vi "ColorDetection2 (2).vi"() -> ()   [LabVIEW 2018]
uses:
  Control 1.ctl
  <vilib>/myRIO/Instrument Drivers/Onboard IO/DIO/typedefs/DIO Reference.ctl
  <vilib>/myRIO/Common/Instrument Driver Framework/Utilities/typedefs/myRIO Generic Hardware Reference.ctl
  <vilib>/myRIO/Common/Instrument Driver Framework/Utilities/typedefs/Hardware Version Enum.ctl
  <vilib>/myRIO/Common/Instrument Driver Framework/Utilities/typedefs/myRIO v1.0 Reference.ctl
  <vilib>/myRIO/Common/Instrument Driver Framework/Utilities/typedefs/Generic FPGA Reference.ctl
  <vilib>/myRIO/Common/Instrument Driver Framework/myRIO v1.0/DIO/typedefs/DIO Channels List.ctl
  <vilib>/myRIO/Common/Instrument Driver Framework/myRIO v1.0/DIO/typedefs/DIO Channels Enum.ctl
  <vilib>/userdefined/High Color/nirio_resource_hc.ctl
  <vilib>/myRIO/Common/Instrument Driver Framework/Utilities/vis/Is FPGA Ref Available.vi
  <vilib>/myRIO/Common/Instrument Driver Framework/myRIO v1.0/DIO/vis/myRIO v1.1 Open DIO.vi
  <vilib>/myRIO/Instrument Drivers/Onboard IO/DIO/vis/Write.vi
  <vilib>/myRIO/Common/Instrument Driver Framework/Utilities/vis/Validate Channels.vi
  <vilib>/myRIO/Common/Instrument Driver Framework/myRIO v1.0/DIO/vis/myRIO v1.0 Reserve DIO.vi
  <vilib>/myRIO/Common/Instrument Driver Framework/myRIO v1.0/UART/vis/myRIO v1.0 Close UART.vi
  <vilib>/myRIO/Common/Instrument Driver Framework/myRIO v1.0/Resource Manager/vis/myRIO v1.0 Reserve Channel List.vi
  <vilib>/myRIO/Common/Instrument Driver Framework/myRIO v1.0/DIO/vis/myRIO v1.0 Build MUX Configuration DIO.vi
  <vilib>/myRIO/Common/Instrument Driver Framework/myRIO v1.0/Resource Manager/vis/myRIO v1.0 Reserve Channel.vi
  <vilib>/myRIO/Common/Instrument Driver Framework/myRIO v1.0/Resource Manager/vis/myRIO v1.0 Unreserve Channel.vi
  <vilib>/myRIO/Common/Instrument Driver Framework/myRIO v1.0/Resource Manager/vis/myRIO v1.0 Create Configuration List.vi
  <vilib>/myRIO/Common/Instrument Driver Framework/myRIO v1.0/Resource Manager/vis/myRIO v1.0 Build Mutex Name.vi
  <vilib>/Utility/VariantDataType/GetNumericInfo.vi
  <vilib>/Utility/error.llb/Error Cluster From Error Code.vi
  <vilib>/myRIO/Common/Instrument Driver Framework/myRIO v1.0/myRIO v1.1 Open.vi
  <vilib>/myRIO/Common/Instrument Driver Framework/Utilities/vis/IO Manager.vi
  <vilib>/myRIO/Common/Instrument Driver Framework/Utilities/vis/Configuration Manager.vi
  <vilib>/myRIO/Common/Instrument Driver Framework/myRIO v1.0/Resource Manager/vis/myRIO v1.0 Configure IO.vi
  <vilib>/myRIO/Common/Instrument Driver Framework/myRIO v1.0/myRIO v1.0 Close.vi
  <vilib>/myRIO/Common/Instrument Driver Framework/myRIO v1.0/DIO/vis/myRIO v1.0 Write DIO.vi
  <vilib>/myRIO/Common/Instrument Driver Framework/Utilities/vis/FPGA Ref Manager.vi
  <vilib>/myRIO/Common/Instrument Driver Framework/myRIO v1.0/myRIO v1.0 Reset FPGA.vi
  <vilib>/myRIO/Common/Instrument Driver Framework/myRIO v1.0/IRQ/vis/myRIO v1.0 IRQ Info FGV.vi
  <vilib>/myRIO/Common/Instrument Driver Framework/myRIO v1.0/IRQ/vis/myRIO v1.0 Timer IRQ Info FGV.vi
  <vilib>/myRIO/Common/Instrument Driver Framework/myRIO v1.0/IRQ/vis/myRIO v1.0 ISR Agent.vi
  <vilib>/myRIO/Express VI/Onboard IO/DO/DO Express VI.xnode
  <vilib>/myRIO/Instrument Drivers/Onboard IO/DIO/vis/myRIO DIO Open.xnode
  <vilib>/myRIO/Instrument Drivers/Utilities/Utilities.lvlib
  <vilib>/myRIO/Instrument Drivers/Onboard IO/DIO/DIO.lvlib
panel:
  out "Time has Elapsed 8":bool caption="Time has Elapsed"
  out "Time has Elapsed 7":bool caption="Time has Elapsed"
  out "Time has Elapsed 6":bool caption="Time has Elapsed"
  out "Time has Elapsed 5":bool caption="Time has Elapsed"
  out "Time has Elapsed 4":bool caption="Time has Elapsed"
  out "Amarillo":bool
  out "Rojo":bool
  out "Azul":bool
  out "Verde":bool
  out "Time has Elapsed 3":bool caption="Time has Elapsed"
  out "Time has Elapsed 2":bool caption="Time has Elapsed"
  out "Time has Elapsed":bool
  out "Negro 3":bool
  out "Amarillo 3":bool
  out "Rojo 3":bool
  out "Azul 3":bool
  out "Verde 3":bool
  out "Color Spectrum 7":dbl[](array[numeric]) format="%.2f"
  out "h3":bool
  out "h2":bool
  out "h1":bool
  out "h0":bool
  out "Negro 1":bool
  out "Amarillo 1":bool
  out "Rojo 1":bool
  out "Azul 1":bool
  out "Verde 1":bool
  out "Negro 2":bool
  out "Amarillo 2":bool
  out "Rojo 2":bool
  out "Azul 2":bool
  out "Verde 2":bool
  out "Color Spectrum 6":dbl[](array[numeric]) format="%.2f"
  out "Color Spectrum 5":dbl[](array[numeric]) format="%.2f"
  out "Negro":bool
  out "Amarillo":bool
  out "Rojo":bool
  out "Azul":bool
  out "Verde":bool
  out "Image Out":T1(plugin-control)
  out "Color Spectrum 4":dbl[](array[numeric]) format="%.2f"
  in  "Stop (F) 2":bool caption="Stop (F)"
  out "Estados":T2
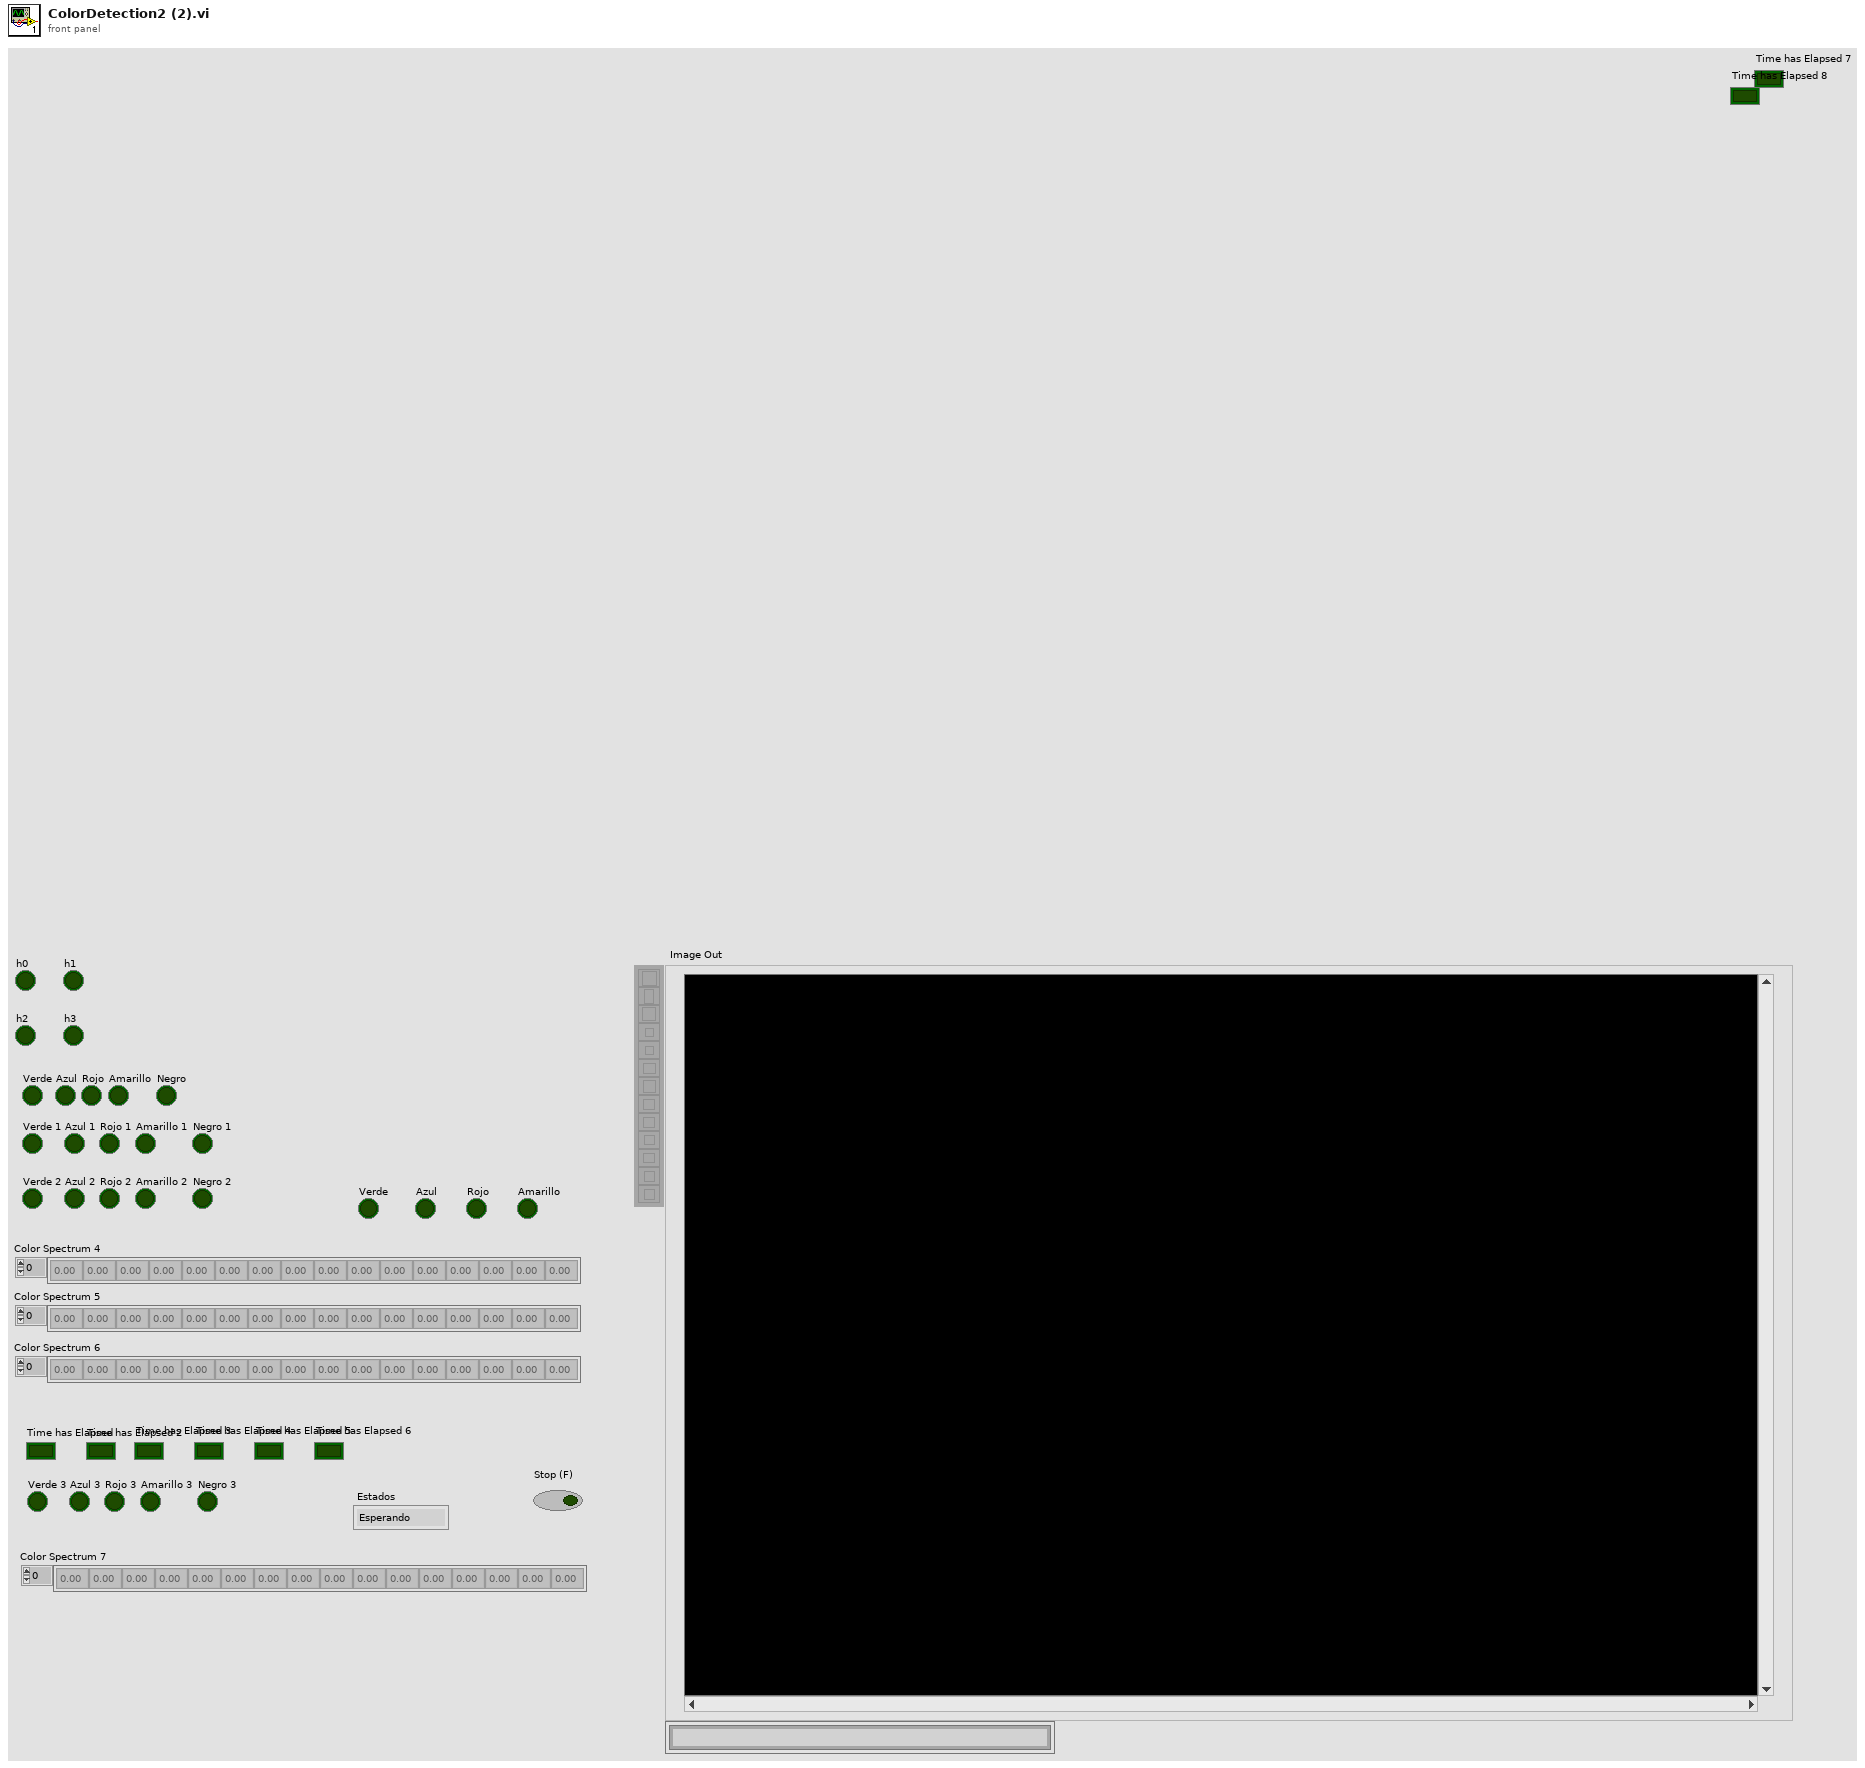
[diagram p1: front panel]
types:
  T1 = typedef "IMAQ Image.ctl" = refnum<image>
  T2 = typedef "Control 1.ctl" = enum16{"Esperando", "Seccion1", "Seccion2", "Seccion3", "Seccion4", "Seccion5", "Seccion6", "Seccion7", "Seccion8", "Seccion9", "Seccion10", "Seccion11", "Seccion12"}
  T3 = typedef "IMAQ Rectangle" = cluster{"Left":i32, "Top":i32, "Right":i32, "Bottom":i32, "Rotation":dbl}
  T4 = typedef "DIO.lvlib/DIO Reference.ctl" = cluster{"myRIO Reference":T5, "DIO Channels List":T9}
  T5 = typedef "myRIO Generic Hardware Reference.ctl" = cluster{"myRIO Model":T6, "myRIO Hardware Reference":T7}
  T6 = typedef "Hardware Version Enum.ctl" = enum16{"Unknown", "myRIO-1900", "myRIO-1950", "roboRIO", "NI ELVIS RIO CM", "ELVIS III"}
  T7 = typedef "myRIO v1.0 Reference.ctl" = cluster{"Generic FPGA Reference":T8, "Allow multiple opens":bool}
  T8 = typedef "Generic FPGA Reference.ctl" = refnum<k20>
  T9 = typedef "DIO Channels List.ctl" = T10[]
  T10 = typedef "DIO Channels Enum.ctl" = enum16{"Not Connected", "C/DIO0", "C/DIO1", "C/DIO2", "C/DIO3", "C/DIO4", "C/DIO5", "C/DIO6", "C/DIO7", "A/DIO0", "A/DIO1", "A/DIO2", "A/DIO3", "A/DIO4", "A/DIO5", "A/DIO6", "A/DIO7", "A/DIO8", "A/DIO9", "A/DIO10", "A/DIO11", "A/DIO12", "A/DIO13", "A/DIO14", "A/DIO15", "A/DIO16", "A/DIO17", "A/DIO18", "A/DIO19", "B/DIO0", "B/DIO1", "B/DIO2", "B/DIO3", "B/DIO4", "B/DIO5", "B/DIO6", "B/DIO7", "B/DIO8", "B/DIO9", "B/DIO10", "B/DIO11", "B/DIO12", "B/DIO13", "B/DIO14", "B/DIO15", "B/DIO16", "B/DIO17", "B/DIO18", "B/DIO19", "LED0", "LED1", "LED2", "LED3", "Button0", "DIO/DIO0", "DIO/DIO1", "DIO/DIO2", "DIO/DIO3", "DIO/DIO4", "DIO/DIO5", "DIO/DIO6", "DIO/DIO7", "DIO/DIO8", "DIO/DIO9", "SPI/CS0", "SPI/CS1", "SPI/CS2", "SPI/CS3", "LED RADIO (Green)", "LED RADIO (Red)", "LED COMM (Green)", "LED COMM (Red)", "LED MODE (Green)", "LED MODE (Red)"}
  T11 = typedef "nirio_resource_hc.ctl" = tag
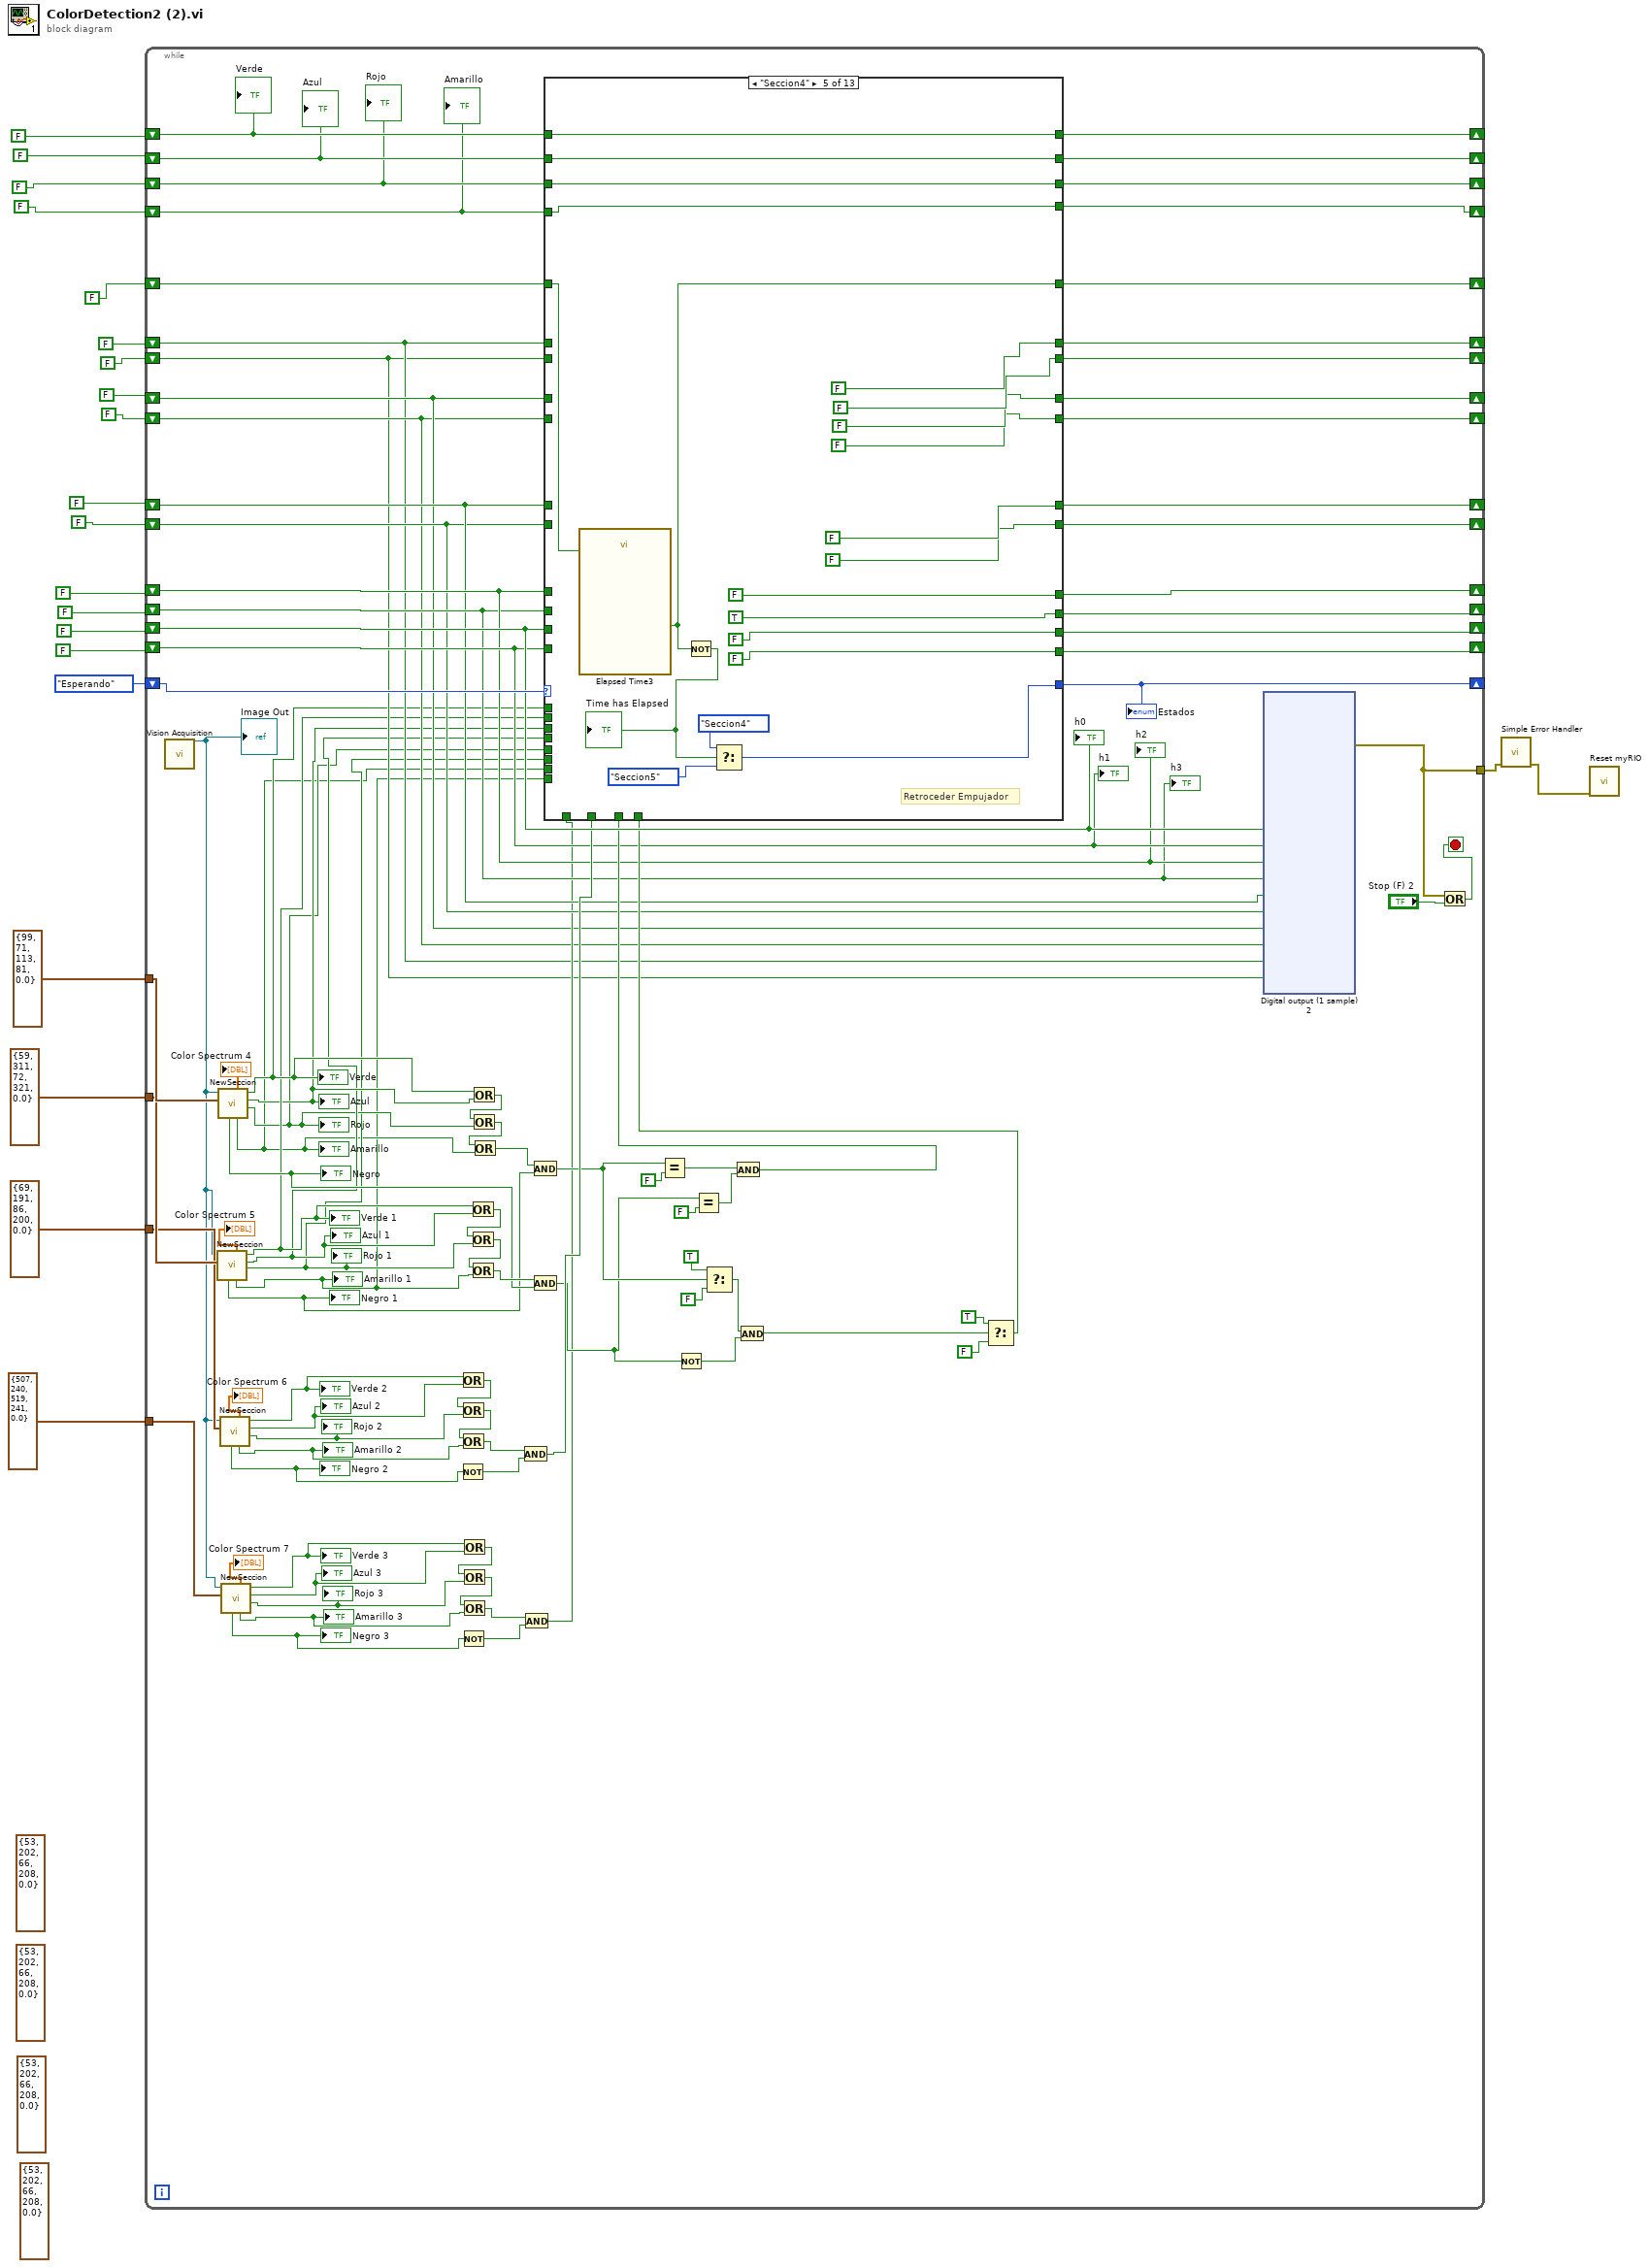
[diagram p0: block diagram]
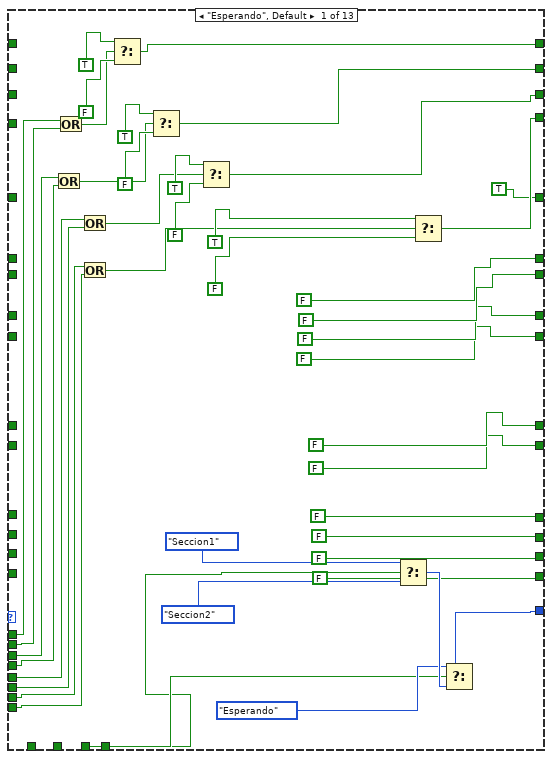
[diagram p2: hidden frame]
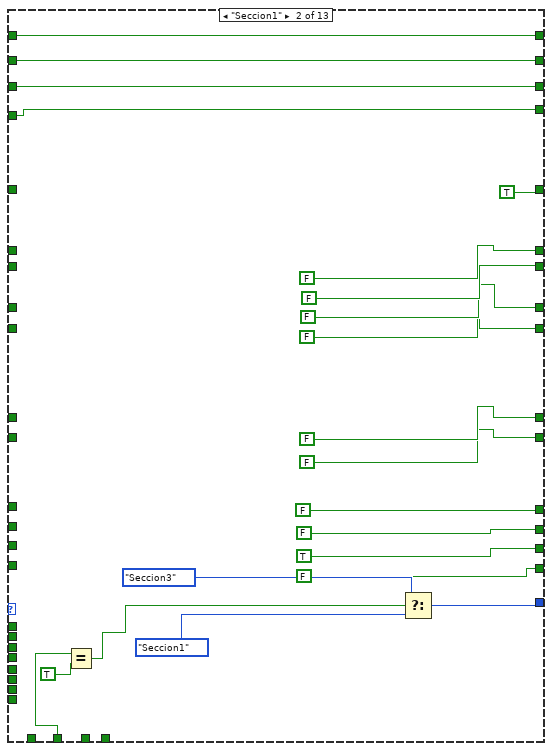
[diagram p3: hidden frame]
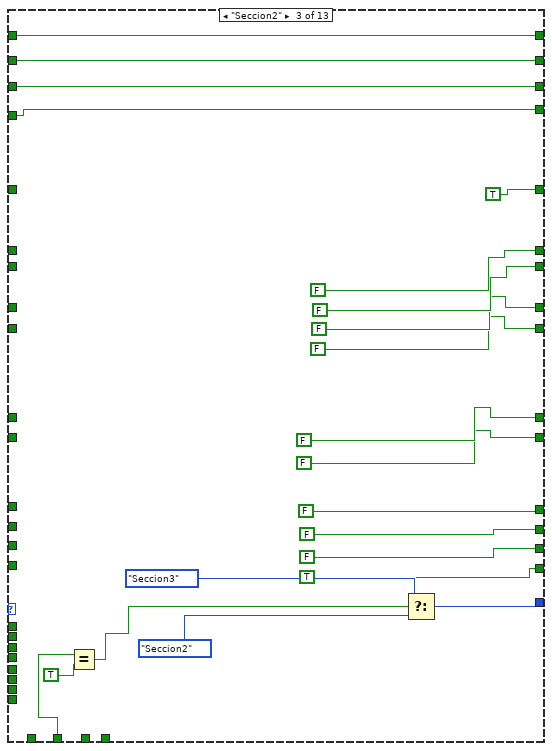
[diagram p4: hidden frame]
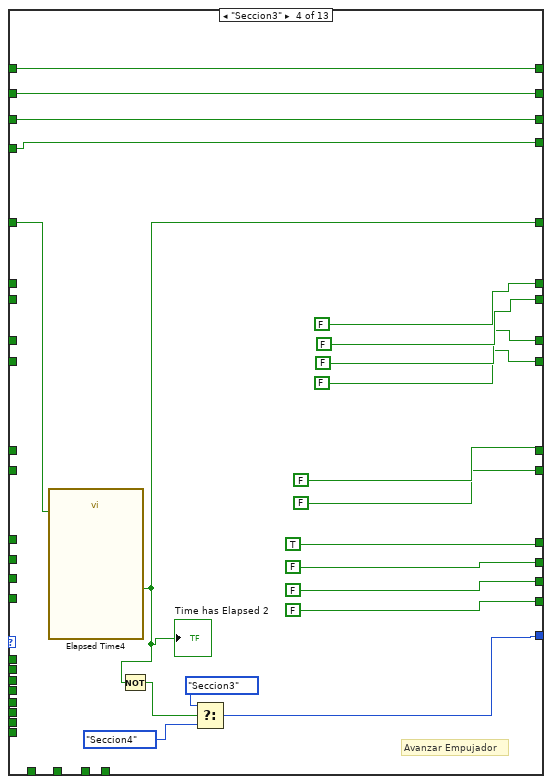
[diagram p5: hidden frame]
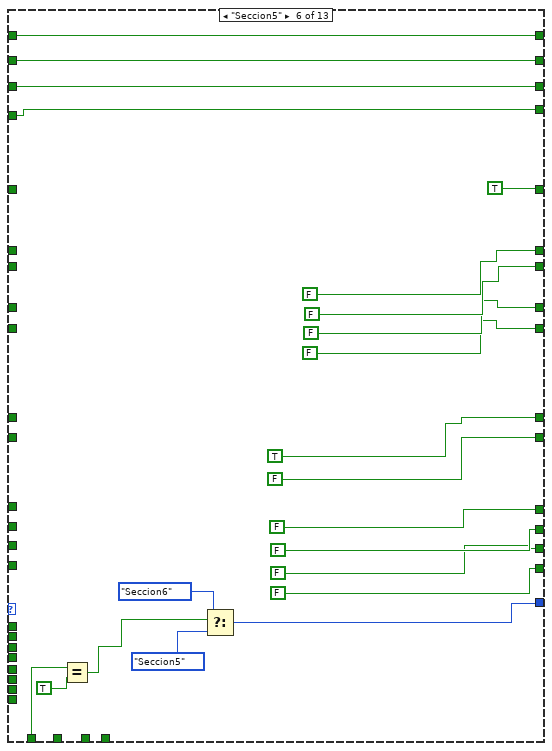
[diagram p6: hidden frame]
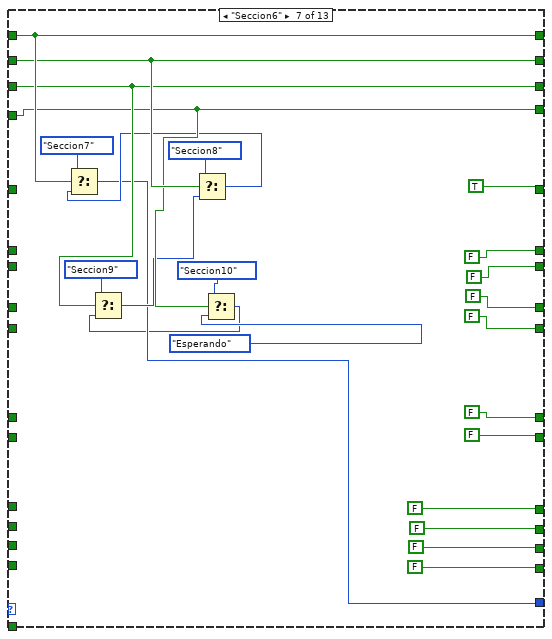
[diagram p7: hidden frame]
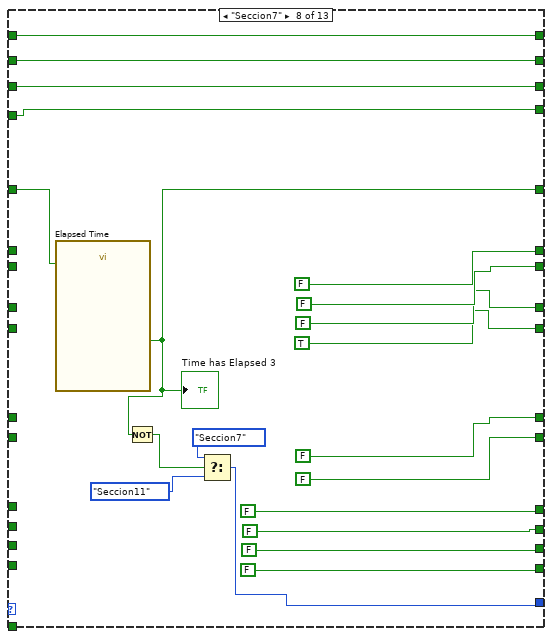
[diagram p8: hidden frame]
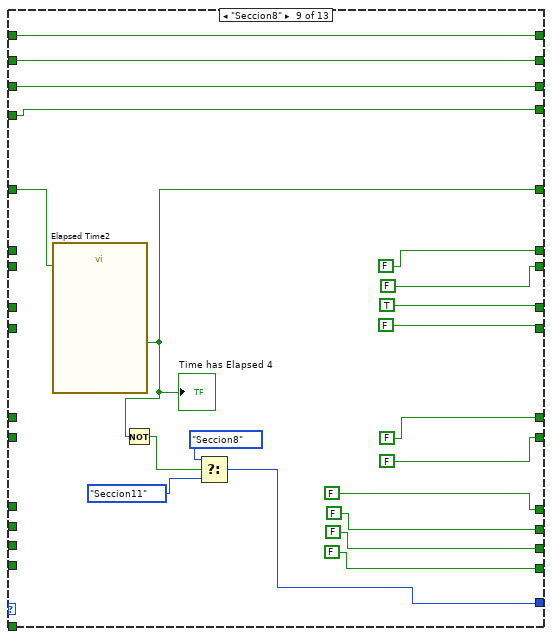
[diagram p9: hidden frame]
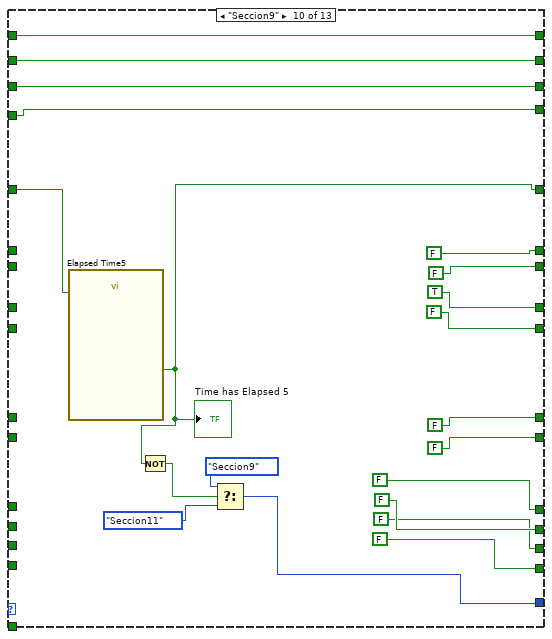
[diagram p10: hidden frame]
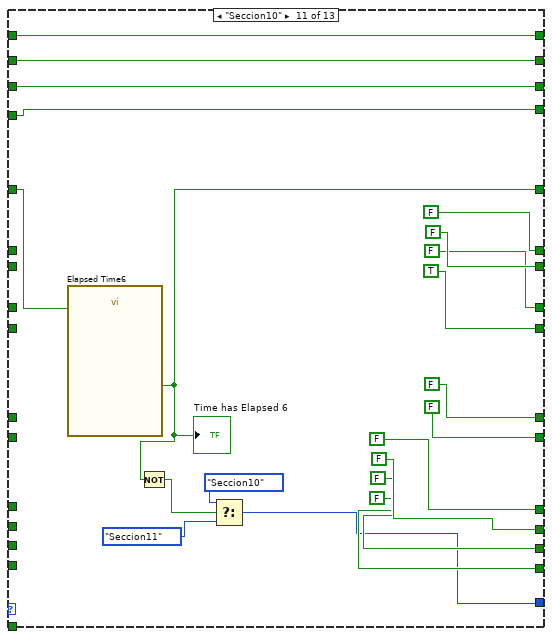
[diagram p11: hidden frame]
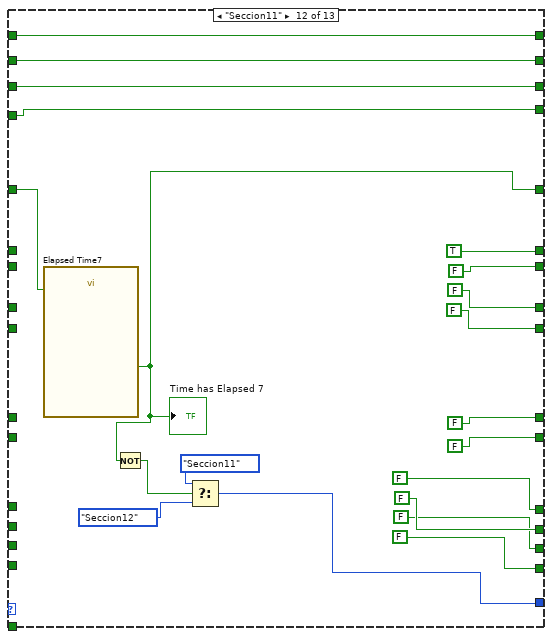
[diagram p12: hidden frame]
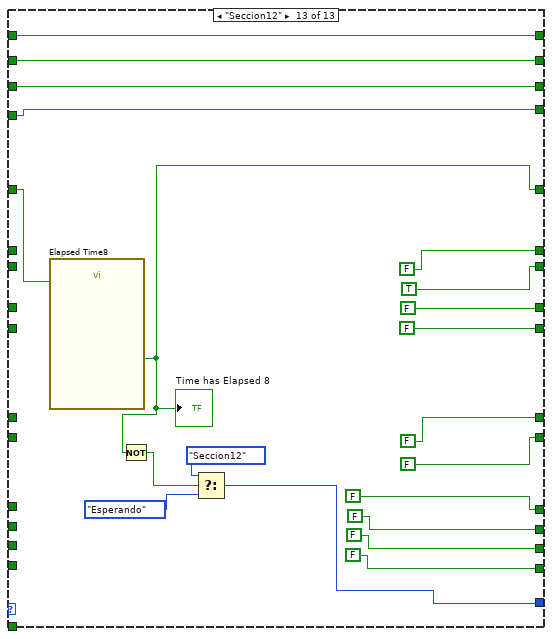
[diagram p13: hidden frame]
diagram:
  (unwired) T3 {"Left"=53, "Top"=202, "Right"=66, "Bottom"=208, "Rotation"=0.0} ("Rectangle")
  (unwired) T3 {"Left"=53, "Top"=202, "Right"=66, "Bottom"=208, "Rotation"=0.0} ("Rectangle")
  (unwired) T3 {"Left"=53, "Top"=202, "Right"=66, "Bottom"=208, "Rotation"=0.0} ("Rectangle")
  (unwired) T3 {"Left"=53, "Top"=202, "Right"=66, "Bottom"=208, "Rotation"=0.0} ("Rectangle")
  n1 = while {
    shift-right: [w112] -> _
    shift-left: Control_1."Esperando" -> [w117]
    shift-right: [w116] -> _
    shift-left: FALSE -> [w68]
    shift-right: [w115] -> _
    shift-left: FALSE -> [w67]
    shift-right: [w114] -> _
    shift-left: FALSE -> [w106]
    shift-right: [w113] -> _
    shift-left: FALSE -> [w69]
    tunnel: T3 {"Left"=99, "Top"=71, "Right"=113, "Bottom"=81, "Rotation"=0.0} ("Rectangle") -> [w108]
    tunnel: T3 {"Left"=59, "Top"=311, "Right"=72, "Bottom"=321, "Rotation"=0.0} ("Rectangle") -> [w105]
    tunnel: T3 {"Left"=69, "Top"=191, "Right"=86, "Bottom"=200, "Rotation"=0.0} ("Rectangle") -> [w104]
    tunnel: [w109] -> w13
    shift-right: [w65] -> _
    shift-left: FALSE -> [w63]
    shift-right: [w64] -> _
    shift-left: FALSE -> [w62]
    tunnel: T3 {"Left"=507, "Top"=240, "Right"=519, "Bottom"=241, "Rotation"=0.0} ("Rectangle") -> [w51]
    shift-right: [w45] -> _
    shift-left: FALSE -> [w43]
    shift-right: [w46] -> _
    shift-left: FALSE -> [w44]
    shift-right: [w47] -> _
    shift-left: FALSE -> [w41]
    shift-right: [w48] -> _
    shift-left: FALSE -> [w42]
    shift-right: [w36] -> _
    shift-left: FALSE -> [w40]
    shift-right: [w35] -> _
    shift-left: FALSE -> [w39]
    shift-right: [w34] -> _
    shift-left: FALSE -> [w38]
    shift-right: [w33] -> _
    shift-left: FALSE -> [w37]
    shift-right: [w23] -> _
    shift-left: FALSE -> [w24]
    stop <- w110 stop-if-true
    n2 = call "Vision Acquisition"() -> ("Image Out"=w50:T1)  [unwired: 25 in, 2 out]
    "Image Out" <- w50
    n3 = call "NewSeccion.vi"("Rectangle"=w105, "Refnum in"=w50) -> ("Rojo"=w27:bool, "Azul"=w29:bool, "Verde"=w31:bool, "Amarillo"=w25:bool, "Color Spectrum"=→"Color Spectrum 5":dbl[], "Negro"=w87:bool)  [unwired: 4 in]
    "Verde 1" <- w31
    "Azul 1" <- w29
    "Rojo 1" <- w27
    "Amarillo 1" <- w25
    "Negro 1" <- w87
    n4 = call "NewSeccion.vi"("Rectangle"=w108, "Refnum in"=w50) -> ("Rojo"=w28:bool, "Azul"=w30:bool, "Verde"=w32:bool, "Amarillo"=w26:bool, "Color Spectrum"=→"Color Spectrum 4":dbl[], "Negro"=w88:bool)  [unwired: 4 in]
    "Verde" <- w32
    "Azul" <- w30
    "Rojo" <- w28
    "Amarillo" <- w26
    "Negro" <- w88
    n5 = call "NewSeccion.vi"("Rectangle"=w104, "Refnum in"=w50) -> ("Rojo"=w97:bool, "Azul"=w96:bool, "Verde"=w98:bool, "Amarillo"=w95:bool, "Color Spectrum"=→"Color Spectrum 6":dbl[], "Negro"=w101:bool)  [unwired: 4 in]
    "Verde 2" <- w98
    "Azul 2" <- w96
    "Rojo 2" <- w97
    "Amarillo 2" <- w95
    "Negro 2" <- w101
    n6 = call "NewSeccion.vi"("Rectangle"=w51, "Refnum in"=w50) -> ("Rojo"=w56:bool, "Azul"=w55:bool, "Verde"=w57:bool, "Amarillo"=w54:bool, "Color Spectrum"=→"Color Spectrum 7":dbl[], "Negro"=w60:bool)  [unwired: 4 in]
    "Verde 3" <- w57
    "Azul 3" <- w55
    "Rojo 3" <- w56
    "Amarillo 3" <- w54
    "Negro 3" <- w60
    n7 = Not(x=w101) -> (.not. x?=w93:bool)
    n8 = Or(x=w98, y=w96) -> (x .or. y?=w100:bool)
    n9 = Or(x=w100, y=w97) -> (x .or. y?=w99:bool)
    n10 = Or(x=w99, y=w95) -> (x .or. y?=w94:bool)
    n11 = Not(x=w60) -> (.not. x?=w52:bool)
    n12 = Or(x=w57, y=w55) -> (x .or. y?=w59:bool)
    n13 = Or(x=w59, y=w56) -> (x .or. y?=w58:bool)
    n14 = Or(x=w58, y=w54) -> (x .or. y?=w53:bool)
    n15 = Or(x=w31, y=w29) -> (x .or. y?=w91:bool)
    n16 = Or(x=w91, y=w27) -> (x .or. y?=w90:bool)
    n17 = Or(x=w90, y=w25) -> (x .or. y?=w89:bool)
    n18 = Or(x=w32, y=w30) -> (x .or. y?=w84:bool)
    n19 = Or(x=w84, y=w28) -> (x .or. y?=w85:bool)
    n20 = Or(x=w85, y=w26) -> (x .or. y?=w86:bool)
    n21 = And(x=w94, y=w93) -> (x .and. y?=w92:bool)
    n22 = And(x=w53, y=w52) -> (x .and. y?=w49:bool)
    n23 = And(x=w86, y=w87) -> (x .and. y?=w75:bool)
    n24 = And(x=w89, y=w88) -> (x .and. y?=w66:bool)
    n25 = Equal?(x=w75, y=FALSE) -> (x = y?=w81:bool)
    n26 = Not(x=w66) -> (.not. x?=w77:bool)
    n27 = Equal?(x=w66, y=FALSE) -> (x = y?=w80:bool)
    n28 = Select(t=TRUE ("y"), s=w75, f=FALSE ("y")) -> (s? t:f=w76:bool)
    n29 = And(x=w81, y=w80) -> (x .and. y?=w71:bool)
    n30 = And(x=w76, y=w77) -> (x .and. y?=w72:bool)
    n31 = Select(t=TRUE, s=w72, f=FALSE) -> (s? t:f=w70:bool)
    n32 = case shown="\"Seccion4\"" w117 {
      tunnel: [FALSE FALSE FALSE TRUE FALSE FALSE FALSE FALSE FALSE FALSE FALSE FALSE FALSE] -> w116
      tunnel: [FALSE FALSE FALSE FALSE TRUE FALSE FALSE FALSE FALSE FALSE FALSE FALSE FALSE] -> w115
      tunnel: [FALSE TRUE FALSE FALSE FALSE FALSE FALSE FALSE FALSE FALSE FALSE FALSE FALSE] -> w114
      tunnel: [FALSE FALSE TRUE FALSE FALSE FALSE FALSE FALSE FALSE FALSE FALSE FALSE FALSE] -> w113
      tunnel: [w193 w220 w241 w259 w279 w302 w309 w333 w353 w373 w393 w411 w433] -> w112
      tunnel: w68 -> [_ _ _ _ _ _ _ _ _ _ _ _ _]
      tunnel: w67 -> [_ _ _ _ _ _ _ _ _ _ _ _ _]
      tunnel: w106 -> [_ _ _ _ _ _ _ _ _ _ _ _ _]
      tunnel: w69 -> [_ _ _ _ _ _ _ _ _ _ _ _ _]
      tunnel: w92 -> [_ w215 w236 _ _ _ _ _ _ _ _ _ _]
      tunnel: w71 -> [w195 _ _ _ _ _ _ _ _ _ _ _ _]
      tunnel: w70 -> [w194 _ _ _ _ _ _ _ _ _ _ _ _]
      tunnel: w63 -> [_ _ _ _ _ _ _ _ _ _ _ _ _]
      tunnel: w62 -> [_ _ _ _ _ _ _ _ _ _ _ _ _]
      tunnel: [FALSE FALSE FALSE FALSE FALSE TRUE FALSE FALSE FALSE FALSE FALSE FALSE FALSE] -> w65
      tunnel: [FALSE FALSE FALSE FALSE FALSE FALSE FALSE FALSE FALSE FALSE FALSE FALSE FALSE] -> w64
      tunnel: w49 -> [_ _ _ _ _ w301 _ _ _ _ _ _ _]
      tunnel: [FALSE FALSE FALSE FALSE FALSE FALSE FALSE FALSE FALSE FALSE FALSE TRUE FALSE] -> w48
      tunnel: [FALSE FALSE FALSE FALSE FALSE FALSE FALSE FALSE FALSE FALSE FALSE FALSE TRUE] -> w47
      tunnel: [FALSE FALSE FALSE FALSE FALSE FALSE FALSE FALSE TRUE TRUE FALSE FALSE FALSE] -> w46
      tunnel: [FALSE FALSE FALSE FALSE FALSE FALSE FALSE TRUE FALSE FALSE TRUE FALSE FALSE] -> w45
      tunnel: w42 -> [_ _ _ _ _ _ _ _ _ _ _ _ _]
      tunnel: w41 -> [_ _ _ _ _ _ _ _ _ _ _ _ _]
      tunnel: w44 -> [_ _ _ _ _ _ _ _ _ _ _ _ _]
      tunnel: w43 -> [_ _ _ _ _ _ _ _ _ _ _ _ _]
      tunnel: w40 -> [_ w208 w229 w251 w271 w290 w320 w340 w370 w380 w400 w420 w450]
      tunnel: w39 -> [_ w207 w228 w250 w270 w289 w314 w339 w369 w379 w399 w419 w449]
      tunnel: w38 -> [_ w206 w227 w249 w269 w288 w313 w338 w368 w378 w398 w418 w448]
      tunnel: w37 -> [_ w205 w226 w248 w268 w287 w312 w337 w367 w377 w397 w417 w447]
      tunnel: [w165 w208 w229 w251 w271 w290 w320 w340 w370 w380 w400 w420 w450] -> w36
      tunnel: [w164 w207 w228 w250 w270 w289 w314 w339 w369 w379 w399 w419 w449] -> w35
      tunnel: [w163 w206 w227 w249 w269 w288 w313 w338 w368 w378 w398 w418 w448] -> w34
      tunnel: [w166 w205 w226 w248 w268 w287 w312 w337 w367 w377 w397 w417 w447] -> w33
      tunnel: w32 -> [w174 _ _ _ _ _ _ _ _ _ _ _ _]
      tunnel: w31 -> [w173 _ _ _ _ _ _ _ _ _ _ _ _]
      tunnel: w30 -> [w172 _ _ _ _ _ _ _ _ _ _ _ _]
      tunnel: w29 -> [w171 _ _ _ _ _ _ _ _ _ _ _ _]
      tunnel: w28 -> [w170 _ _ _ _ _ _ _ _ _ _ _ _]
      tunnel: w27 -> [w169 _ _ _ _ _ _ _ _ _ _ _ _]
      tunnel: w26 -> [w168 _ _ _ _ _ _ _ _ _ _ _ _]
      tunnel: w25 -> [w167 _ _ _ _ _ _ _ _ _ _ _ _]
      tunnel: w24 -> [_ _ _ w247 w267 _ _ w331 w352 w372 w391 w412 w431]
      tunnel: [TRUE TRUE TRUE w246 w266 TRUE TRUE w332 w351 w371 w392 w413 w432] -> w23
      frame "Esperando", Default {
        n33 = Or(x=w172, y=w171) -> (x .or. y?=w177:bool)
        n34 = Or(x=w174, y=w173) -> (x .or. y?=w178:bool)
        n35 = Or(x=w170, y=w169) -> (x .or. y?=w176:bool)
        n36 = Or(x=w168, y=w167) -> (x .or. y?=w175:bool)
        n37 = Select(t=TRUE, s=w178, f=FALSE) -> (s? t:f=w165:bool)
        n38 = Select(t=TRUE, s=w177, f=FALSE) -> (s? t:f=w164:bool)
        n39 = Select(t=TRUE, s=w176, f=FALSE) -> (s? t:f=w163:bool)
        n40 = Select(t=Control_1."Seccion1", s=w194, f=Control_1."Seccion2") -> (s? t:f=w201:T2)
        n41 = Select(t=TRUE, s=w175, f=FALSE) -> (s? t:f=w166:bool)
        n42 = Select(t=Control_1."Esperando", s=w195, f=w201) -> (s? t:f=w193:T2)
      }
      frame "Seccion1" {
        n43 = Equal?(x=w215, y=TRUE) -> (x = y?=w223:bool)
        n44 = Select(t=Control_1."Seccion3", s=w223, f=Control_1."Seccion1") -> (s? t:f=w220:T2)
      }
      frame "Seccion2" {
        n45 = Equal?(x=w236, y=TRUE) -> (x = y?=w244:bool)
        n46 = Select(t=Control_1."Seccion3", s=w244, f=Control_1."Seccion2") -> (s? t:f=w241:T2)
      }
      frame "Seccion3" {
        # "Avanzar Empujador"
        n47 = call "Elapsed Time4"("Reset"=w247) -> ("Time has Elapsed"=w246:bool)  [unwired: 11 in, 7 out]
        "Time has Elapsed 2" <- w246
        n48 = Not(x=w246) -> (.not. x?=w256:bool)
        n49 = Select(t=Control_1."Seccion3", s=w256, f=Control_1."Seccion4") -> (s? t:f=w259:T2)
      }
      frame "Seccion4" {
        # "Retroceder Empujador"
        n50 = call "Elapsed Time3"("Reset"=w267) -> ("Time has Elapsed"=w266:bool)  [unwired: 11 in, 7 out]
        n51 = Not(x=w266) -> (.not. x?=w276:bool)
        "Time has Elapsed" <- w276
        n52 = Select(t=Control_1."Seccion4", s=w276, f=Control_1."Seccion5") -> (s? t:f=w279:T2)
      }
      frame "Seccion5" {
        n53 = Equal?(x=w301, y=TRUE) -> (x = y?=w305:bool)
        n54 = Select(t=Control_1."Seccion6", s=w305, f=Control_1."Seccion5") -> (s? t:f=w302:T2)
      }
      frame "Seccion6" {
        n55 = Select(t=Control_1."Seccion10", s=w312, f=Control_1."Esperando") -> (s? t:f=w308:T2)
        n56 = Select(t=Control_1."Seccion9", s=w313, f=w308) -> (s? t:f=w310:T2)
        n57 = Select(t=Control_1."Seccion8", s=w314, f=w310) -> (s? t:f=w311:T2)
        n58 = Select(t=Control_1."Seccion7", s=w320, f=w311) -> (s? t:f=w309:T2)
      }
      frame "Seccion7" {
        n59 = call "Elapsed Time"("Reset"=w331) -> ("Time has Elapsed"=w332:bool)  [unwired: 11 in, 7 out]
        "Time has Elapsed 3" <- w332
        n60 = Not(x=w332) -> (.not. x?=w334:bool)
        n61 = Select(t=Control_1."Seccion7", s=w334, f=Control_1."Seccion11") -> (s? t:f=w333:T2)
      }
      frame "Seccion8" {
        n62 = call "Elapsed Time2"("Reset"=w352) -> ("Time has Elapsed"=w351:bool)  [unwired: 11 in, 7 out]
        "Time has Elapsed 4" <- w351
        n63 = Not(x=w351) -> (.not. x?=w354:bool)
        n64 = Select(t=Control_1."Seccion8", s=w354, f=Control_1."Seccion11") -> (s? t:f=w353:T2)
      }
      frame "Seccion9" {
        n65 = call "Elapsed Time5"("Reset"=w372) -> ("Time has Elapsed"=w371:bool)  [unwired: 11 in, 7 out]
        "Time has Elapsed 5" <- w371
        n66 = Not(x=w371) -> (.not. x?=w374:bool)
        n67 = Select(t=Control_1."Seccion9", s=w374, f=Control_1."Seccion11") -> (s? t:f=w373:T2)
      }
      frame "Seccion10" {
        n68 = call "Elapsed Time6"("Reset"=w391) -> ("Time has Elapsed"=w392:bool)  [unwired: 11 in, 7 out]
        "Time has Elapsed 6" <- w392
        n69 = Not(x=w392) -> (.not. x?=w394:bool)
        n70 = Select(t=Control_1."Seccion10", s=w394, f=Control_1."Seccion11") -> (s? t:f=w393:T2)
      }
      frame "Seccion11" {
        n71 = call "Elapsed Time7"("Reset"=w412) -> ("Time has Elapsed"=w413:bool)  [unwired: 11 in, 7 out]
        "Time has Elapsed 7" <- w413
        n72 = Not(x=w413) -> (.not. x?=w414:bool)
        n73 = Select(t=Control_1."Seccion11", s=w414, f=Control_1."Seccion12") -> (s? t:f=w411:T2)
      }
      frame "Seccion12" {
        n74 = call "Elapsed Time8"("Reset"=w431) -> ("Time has Elapsed"=w432:bool)  [unwired: 11 in, 7 out]
        "Time has Elapsed 8" <- w432
        n75 = Not(x=w432) -> (.not. x?=w434:bool)
        n76 = Select(t=Control_1."Seccion12", s=w434, f=Control_1."Esperando") -> (s? t:f=w433:T2)
      }
    }
    "Estados" <- w112
    n77 = xnode "Digital output (1 sample) 2"("h0 (B/DIO1 (Pin 13))"=w106, "h1 (B/DIO0 (Pin 11))"=w69, "h2 (B/DIO2 (Pin 15))"=w68, "h3 (B/DIO3 (Pin 17))"=w67, "h4 (B/DIO4 (Pin 19))"=w63, "h5 (B/DIO5 (Pin 21))"=w62, "h6 (B/DIO6 (Pin 23))"=w44, "h7 (B/DIO7 (Pin 25))"=w43, "h8 (B/DIO8 (Pin 27))"=w42, "h9 (B/DIO9 (Pin 29))"=w41) -> ("error out"=w109:errorcluster)  [unwired: 1 in]
    n78 = Or(x=w109, y="Stop (F) 2") -> (x .or. y?=w110:bool)
    "h0" <- w106
    "h1" <- w69
    "h2" <- w68
    "h3" <- w67
    "Verde" <- w40
    "Azul" <- w39
    "Rojo" <- w38
    "Amarillo" <- w37
  }
  n79 = call <vilib>:"Simple Error Handler.vi"("error in (no error)"=w13) -> ("error out"=w14:errorcluster)  [unwired: 4 in, 4 out]
  n80 = call <vilib>:"Reset myRIO.vi"("error in (no error)"=w14) -> ()  [unwired: 10 in, 1 out]
